vi "Xml_UpdateValueByName.vi"(6 "offset (0)":i32, 8 "error in (no error)":errorcluster, 9 "New Value":string, 10 "TagName":string, 11 "XML String":string) -> (0 "error out":errorcluster, 3 "XML String Out":string)   [LabVIEW 2021, in "XML.lvlib"]
uses:
  XML.lvlib
panel:
  out "match substring":string
  out "offset past match":i32
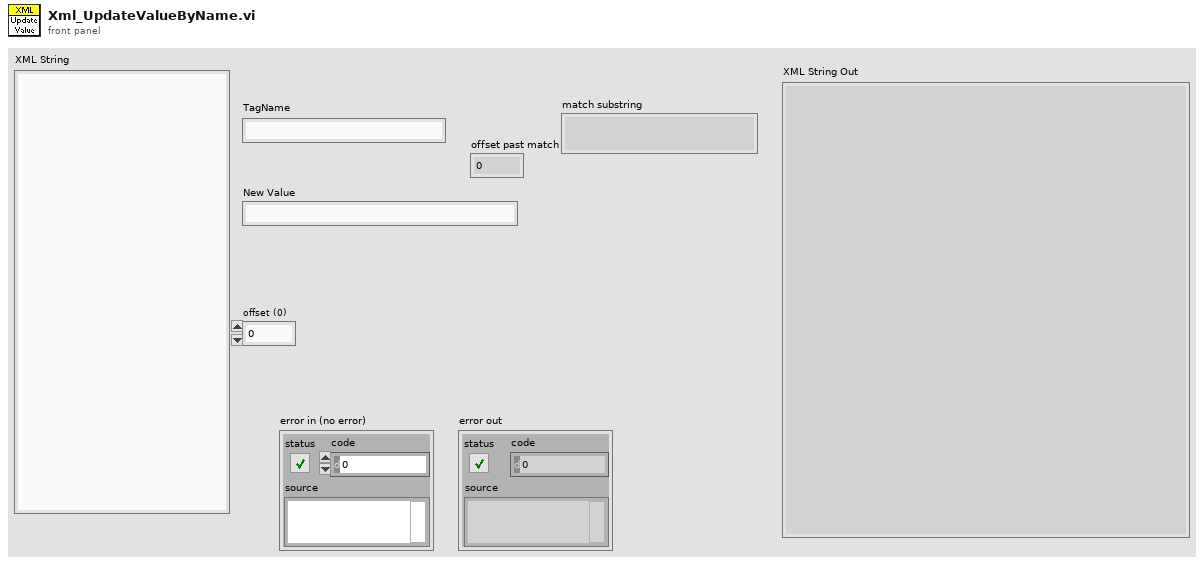
[diagram p1: front panel]
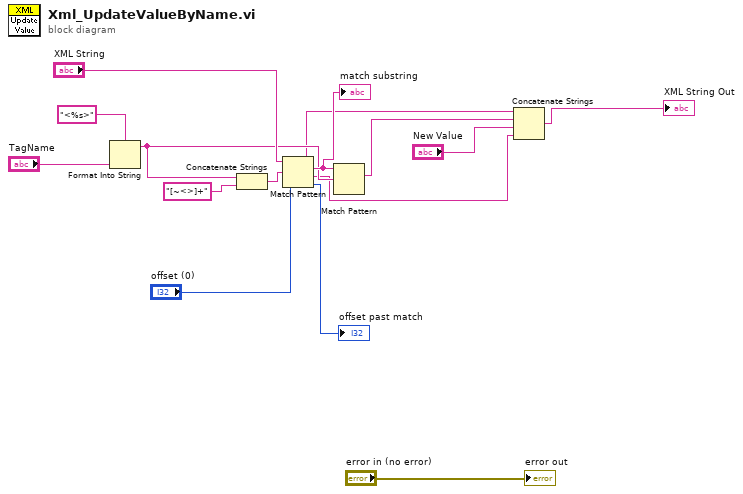
[diagram p0: block diagram]
diagram:
  n1 = Format Into String(format string="<%s>" ("regular expression"), "TagName") -> (resulting string=w9:string)  [unwired: 2 in, 1 out]
  n2 = Concatenate Strings(w9, "[~<>]+" ("string")) -> (w15:string)
  n3 = Match Pattern(string="XML String", regular expression=w15, offset (0)="offset (0)") -> (before substring=w6:string, match substring=w13:string, after substring=w4:string, offset past match=→"offset past match":i32)
  "match substring" <- w13
  n4 = Match Pattern(string=w13, regular expression=w9) -> (match substring=w5:string)  [unwired: 1 in, 3 out]
  n5 = Concatenate Strings(w6, w5, "New Value", w4) -> (→"XML String Out":string)
  "error out" <- "error in (no error)"
